vi "Lab Arreglos-5.vi"() -> ()   [LabVIEW 2018]
panel:
  out "Array":void[][](array[numeric])
  in  "stop":bool
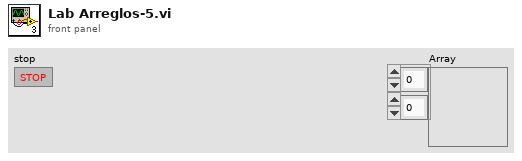
[diagram p1: front panel]
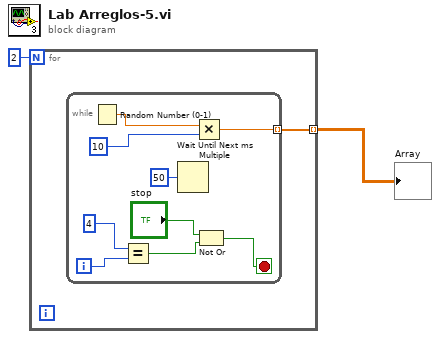
[diagram p0: block diagram]
diagram:
  n1 = for {
    N: 2 -> [_]
    tunnel: [w3] -> w1 mode=indexing
    n2 = while {
      tunnel: [w9] -> w3 mode=indexing
      i -> [w8]
      stop <- w4 stop-if-true
      n3 = Random Number (0-1)() -> (number: 0 to 1=w12:dbl)
      n4 = Equal?(x=4, y=w8) -> (x = y?=w6:bool)
      n5 = Wait Until Next ms Multiple(millisecond multiple=u32 50) -> ()  [unwired: 1 out]
      n6 = Multiply(x=w12, y=10) -> (x*y=w9:dbl)
      n7 = Not Or(1:w6, 2:"stop") -> (0:w4:bool)
    }
  }
  "Array" <- w1
